vi "AI Referenece.vi"(8 "error in (no error)":errorcluster, 11 "Child Refs":T1[](array[typedef]) format="%.0x") -> (0 "error in (no error) 2":errorcluster, 1 "AI Refs":T1[](array[typedef]) format="%.0x", 3 "AI Refs":T2(array[cluster]) {"VS Refs" format="%.0x"})   [LabVIEW 2021, in "DAQ Analog InOut System Explorer.lvlib"]
uses:
  <vilib>/NI VeriStand/Custom Device API/Custom Device Item Ref.ctl
  DAQ Analog InOut System Explorer.lvlib
  <vilib>/NI VeriStand/Custom Device API/Custom Device API.lvlib
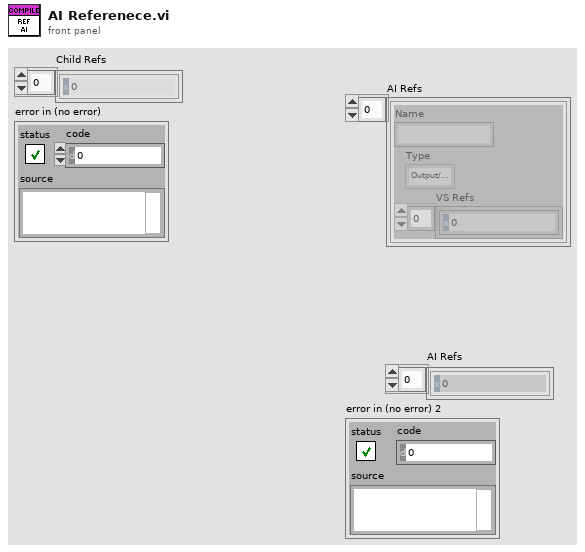
[diagram p1: front panel]
types:
  T1 = typedef "Custom Device API.lvlib/Custom Device Item Ref.ctl" = u64
  T2 = cluster{"Name":string, "Type":enum16{"Output/Write", "Input/Read", "Input/ReadWrite"}, "VS Refs":T1[]}[]
  T3 = enum16{"Output/Write", "Input/Read", "Input/ReadWrite"}
  T4 = cluster{"Name":string, "Type":enum16{"Output/Write", "Input/Read", "Input/ReadWrite"}, "VS Refs":T1[]}
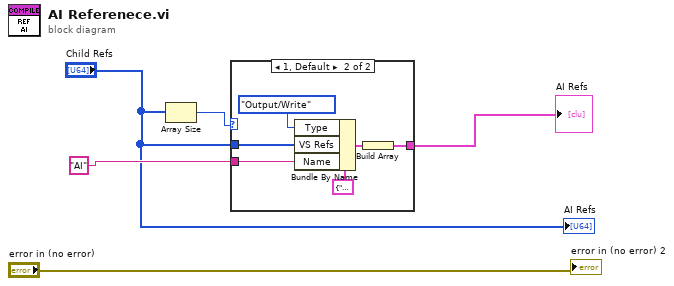
[diagram p0: block diagram]
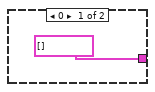
[diagram p2: hidden frame]
diagram:
  n1 = Array Size(array="Child Refs") -> (size(s)=w5:i32)
  n2 = case shown="1, Default" w5 {
    tunnel: "Child Refs" -> [_ w10]
    tunnel: [T2 [] w8] -> w3
    tunnel: "AI" ("Name") -> [_ w7]
    frame 0 {
    }
    frame 1, Default {
      n3 = Bundle By Name(cluster=T4 {"Name"="", "Type"=enum."Output/Write", "VS Refs"=[]} ("Group"), "Type"=T3."Output/Write", "VS Refs"=w10, "Name"=w7) -> (w9:T4)
      n4 = Build Array(w9) -> (w8:T2)
    }
  }
  "AI Refs" <- w3
  "AI Refs" <- "Child Refs"
  "error in (no error) 2" <- "error in (no error)"
